vi "EDL Cap.vi"(0 "T":dbl, 1 "er":dbl, 2 "z":dbl, 3 "Co; miliMolar (moles/m3)":dbl, 4 "Co nM-M":dbl, 5 "V  nV-m V-V":dbl, 6 "V zeta":dbl, 8 "# of CNTs in 1 NS":dbl, 10 "Surface Area of 1 CNT":dbl) -> (7 "V_Zeta":dbl, 12 "eo; Permitivity of Free Space 2":dbl, 14 "N_a; Avagadro no":dbl=1.38064852e-23, 15 "C in M":dbl, 16 "eo; Permitivity of Free Space":dbl=8.85418782e-12, 17 "C_EDL/ 1 NS":dbl, 18 "k; Boltzmann Constant":dbl=1.38064852e-23, 19 "C_EDL/ 1 CNT":dbl, 20 "F=eN_a":dbl, 21 "R=kN_a":dbl, 22 "c; Charge on e":dbl=1.6021766208e-19, 23 "C EDL by d with Cosh Factor":dbl format="%#_6e", 24 "C EDL by d":dbl, 25 "d; EDL Length":dbl, 26 "C_EDL/ A":dbl format="%#_6e")   [LabVIEW 2020]
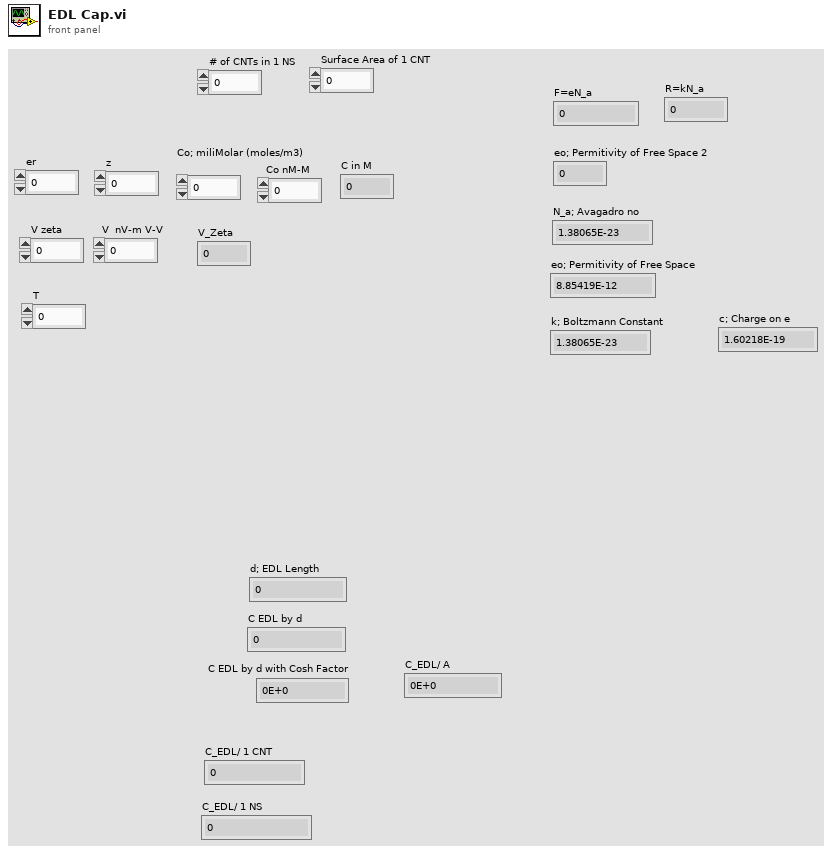
[diagram p1: front panel]
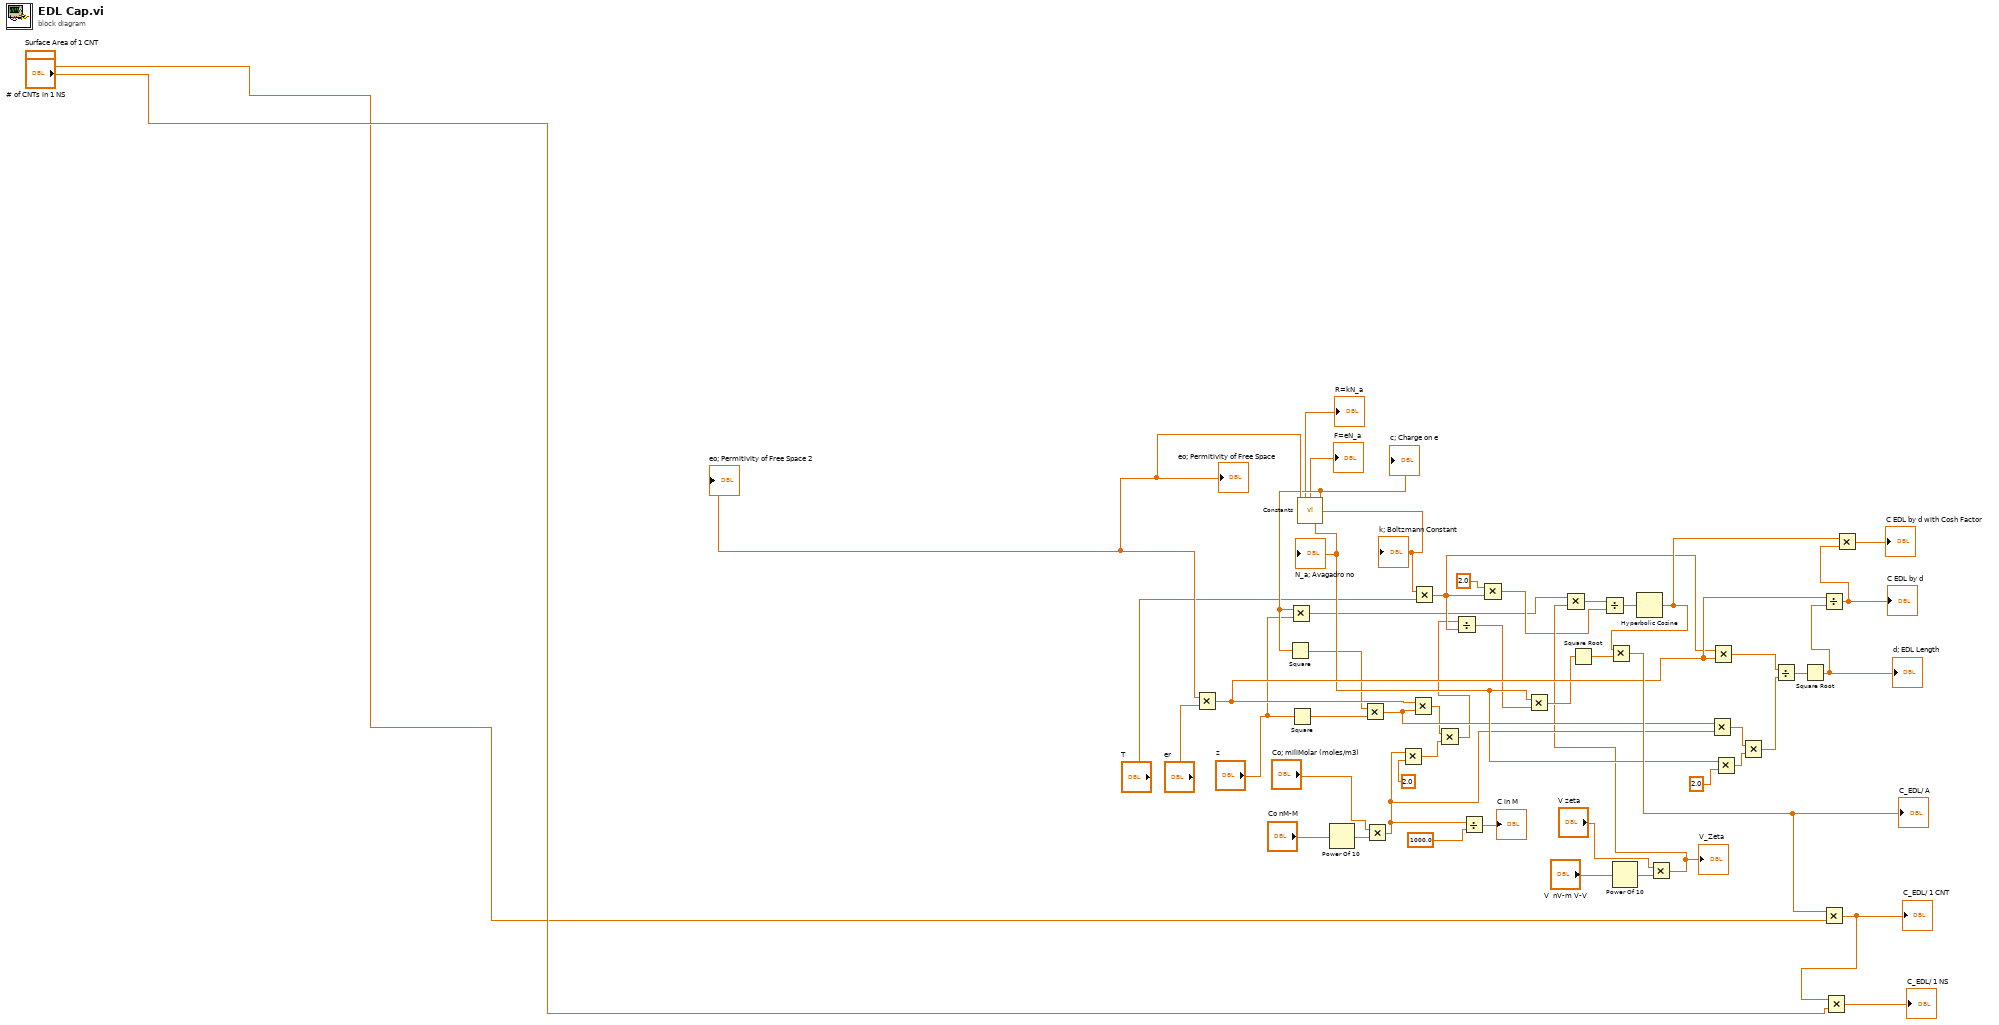
[diagram p0: block diagram]
diagram:
  n1 = Square(x="z") -> (x^2=w1:dbl)
  n2 = call "Constants.vi"() -> ("eo; Permitivity of Free Space"=w41:dbl, "c; Charge on e"=w30:dbl, "k; Boltzmann Constant"=w29:dbl, "R=kN_a"=→"R=kN_a":dbl, "F=eN_a"=→"F=eN_a":dbl, "N_a; Avagadro no"=w35:dbl)  [unwired: 10 in]
  "eo; Permitivity of Free Space" <- w41
  "k; Boltzmann Constant" <- w29
  "c; Charge on e" <- w30
  "N_a; Avagadro no" <- w35
  "eo; Permitivity of Free Space 2" <- w41
  n3 = Multiply(x=w41, y="er") -> (x*y=w43:dbl)
  n4 = Square(x=w30) -> (x^2=w2:dbl)
  n5 = Multiply(x=w30, y="z") -> (x*y=w16:dbl)
  n6 = Power Of 10(x="Co nM-M") -> (10^x=w8:dbl)
  n7 = Multiply(x=w2, y=w1) -> (x*y=w31:dbl)
  n8 = Multiply(x="Co; miliMolar (moles/m3)", y=w8) -> (x*y=w32:dbl)
  n9 = Multiply(x=w32, y=2.0) -> (x*y=w5:dbl)
  n10 = Multiply(x=w43, y=w31) -> (x*y=w6:dbl)
  n11 = Multiply(x=w29, y="T") -> (x*y=w33:dbl)
  n12 = Multiply(x=w6, y=w5) -> (x*y=w13:dbl)
  n13 = Divide(x=w13, y=w33) -> (x/y=w24:dbl)
  n14 = Divide(x=w32, y=1000.0 ("x")) -> (x/y=→"C in M":dbl)
  n15 = Multiply(x=2.0, y=w33) -> (x*y=w18:dbl)
  n16 = Multiply(x=w35, y=w24) -> (x*y=w26:dbl)
  n17 = Square Root(x=w26) -> (sqrt(x)=w25:dbl)
  n18 = Power Of 10(x="V  nV-m V-V") -> (10^x=w20:dbl)
  n19 = Multiply(x="V zeta", y=w20) -> (x*y=w22:dbl)
  "V_Zeta" <- w22
  n20 = Multiply(x=w16, y=w22) -> (x*y=w17:dbl)
  n21 = Divide(x=w17, y=w18) -> (x/y=w19:dbl)
  n22 = Hyperbolic Cosine(1:w19) -> (0:w44:dbl)
  n23 = Multiply(x=w44, y=w25) -> (x*y=w47:dbl)
  "C_EDL/ A" <- w47
  n24 = Multiply(x=w31, y=w32) -> (x*y=w37:dbl)
  n25 = Multiply(x=w33, y=w43) -> (x*y=w38:dbl)
  n26 = Multiply(x=w35, y=2.0) -> (x*y=w36:dbl)
  n27 = Multiply(x=w37, y=w36) -> (x*y=w39:dbl)
  n28 = Divide(x=w38, y=w39) -> (x/y=w40:dbl)
  n29 = Square Root(x=w40) -> (sqrt(x)=w42:dbl)
  "d; EDL Length" <- w42
  n30 = Divide(x=w43, y=w42) -> (x/y=w45:dbl)
  "C EDL by d" <- w45
  n31 = Multiply(x=w47, y="Surface Area of 1 CNT") -> (x*y=w50:dbl)
  "C_EDL/ 1 CNT" <- w50
  n32 = Multiply(x=w50, y="# of CNTs in 1 NS") -> (x*y=→"C_EDL/ 1 NS":dbl)
  n33 = Multiply(x=w44, y=w45) -> (x*y=→"C EDL by d with Cosh Factor":dbl)
